vi "Get All Artists.vi"(8 "error in (no error)":errorcluster, 11 "MusicLibrary in":refnum<class "MusicLibrary.lvclass">) -> (0 "error out":errorcluster, 2 "Artist Library":refnum<class "MusicLibrary.lvclass">, 3 "MusicLibrary out":refnum<class "MusicLibrary.lvclass">)   [LabVIEW 2015, in "MusicLibrary.lvclass"]
uses:
  MusicLibrary.lvclass
  Song/Song.lvclass/Song.ctl
  MusicElementLibrary.lvclass/MusicElementLibrary.ctl
  SongLibrary/SongLibrary.lvclass
  MusicElement.lvclass
  Song/Song.lvclass
  MusicElementLibrary.lvclass
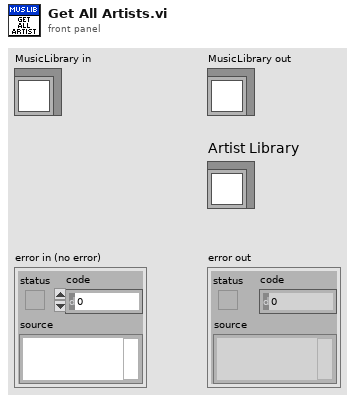
[diagram p1: front panel]
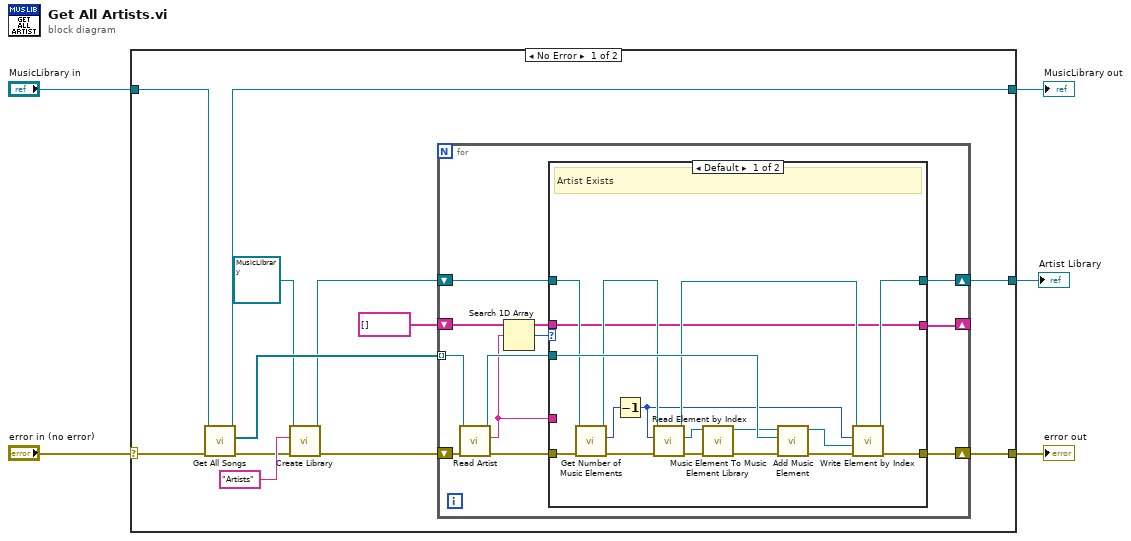
[diagram p0: block diagram]
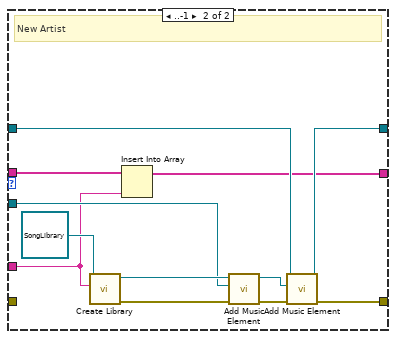
[diagram p2: hidden frame]
diagram:
  n1 = case shown="No Error" "error in (no error)" {
    selector: "error in (no error)" -> [w17 w59]
    tunnel: [w7 w59] -> w4
    tunnel: [w15 w58] -> w2
    tunnel: "MusicLibrary in" -> [w16 w58]
    tunnel: [w8 _] -> w1
    frame No Error {
      n2 = call "Get All Songs.vi"("error in (no error)"=w17, "MusicLibrary in"=w16) -> ("error out"=w9:errorcluster, "Songs"=w14:refnum<class "Song.lvclass">[], "MusicLibrary out"=w15:refnum<class "MusicLibrary.lvclass">)  [unwired: 7 in]
      n3 = call "Create Library.vi"("error in (no error)"=w9, "Name"="Artists", "MusicElementLibrary in"=refnum<class "MusicLibrary.lvclass"> refnum ("MusicLibrary.lvclass")) -> ("error out"=w11:errorcluster, "MusicElementLibrary out"=w12:refnum<class "MusicLibrary.lvclass">)  [unwired: 7 in]
      n4 = for {
        shift-right: [w24] -> w7
        shift-left: w11 -> [w28]
        tunnel: w14 -> [w27] mode=indexing
        shift-right: [w25] -> w8
        shift-left: w12 -> [w23]
        shift-right: [w18] -> _
        shift-left: string[] [] -> [w20]
        n5 = call "Read Artist.vi"("error in (no error)"=w28, "Song in"=w27) -> ("error out"=w22:errorcluster, "Artist"=w19:string, "Song out"=w26:refnum<class "Song.lvclass">)  [unwired: 7 in]
        n6 = Search 1D Array(1D array=w20, element=w19) -> (index of element=w21:i32)  [unwired: 1 in]
        n7 = case shown="Default" w21 {
          tunnel: w23 -> [w44 w53]
          tunnel: w19 -> [_ w47]
          tunnel: w26 -> [w45 w55]
          tunnel: [w32 w50] -> w24
          tunnel: [w31 w52] -> w25
          tunnel: w22 -> [w30 _]
          tunnel: w20 -> [w29 w48]
          tunnel: [w29 w46] -> w18
          frame Default {
            # "Artist Exists"
            n8 = call "Get Number of Music Elements.vi"("error in (no error)"=w30, "MusicElementLibrary in"=w44) -> ("error out"=w43:errorcluster, "Size"=w42:i32, "MusicElementLibrary out"=w41:refnum<class "MusicLibrary.lvclass">)  [unwired: 7 in]
            n9 = Decrement(x=w42) -> (x-1=w33:i32)
            n10 = call "Read Element by Index.vi"("error in (no error)"=w43, "index"=w33, "MusicElementLibrary in"=w41) -> ("error out"=w40:errorcluster, "MusicElement.lvclass"=w39:refnum<class "MusicElement.lvclass">, "MusicElementLibrary out"=w37:refnum<class "MusicLibrary.lvclass">)  [unwired: 5 in, 1 out]
            n11 = call "Music Element To Music Element Library.vi"("error in (no error)"=w40, "MusicElement"=w39) -> ("error out"=w36:errorcluster, "MusicElementLibrary out"=w38:refnum<class "MusicElementLibrary.lvclass">)  [unwired: 8 in]
            n12 = call "Add Music Element.vi"("error in (no error)"=w36, "MusicElement"=w45, "MusicElementLibrary in"=w38) -> ("error out"=w35:errorcluster, "MusicElementLibrary out"=w34:refnum<class "MusicElementLibrary.lvclass">)  [unwired: 7 in]
            n13 = call "Write Element by Index.vi"("error in (no error)"=w35, "MusicElement.lvclass"=w34, "index"=w33, "MusicElementLibrary in"=w37) -> ("error out"=w32:errorcluster, "MusicElementLibrary out"=w31:refnum<class "MusicLibrary.lvclass">)  [unwired: 5 in, 1 out]
          }
          frame ..-1 {
            # "New Artist"
            n14 = call "Create Library.vi"("Name"=w47, "MusicElementLibrary in"=refnum<class "SongLibrary.lvclass"> refnum ("SongLibrary.lvclass")) -> ("error out"=w57:errorcluster, "MusicElementLibrary out"=w56:refnum<class "SongLibrary.lvclass">)  [unwired: 8 in]
            n15 = Insert Into Array(array=w48, new element=w47) -> (w46:string[])  [unwired: 1 in]
            n16 = call "Add Music Element.vi"("error in (no error)"=w57, "MusicElement"=w55, "MusicElementLibrary in"=w56) -> ("error out"=w54:errorcluster, "MusicElementLibrary out"=w51:refnum<class "SongLibrary.lvclass">)  [unwired: 7 in]
            n17 = call "Add Music Element.vi"("error in (no error)"=w54, "MusicElement"=w51, "MusicElementLibrary in"=w53) -> ("error out"=w50:errorcluster, "MusicElementLibrary out"=w52:refnum<class "MusicLibrary.lvclass">)  [unwired: 7 in]
          }
        }
      }
    }
    frame Error {
    }
  }
  "error out" <- w4
  "MusicLibrary out" <- w2
  "Artist Library" <- w1
